vi "VIPM Artifactory Repository.vi"() -> ()   [LabVIEW 2021]
uses:
  Artifactory/Status -- cluster.ctl
  Artifactory/Public Events -- cluster.ctl
  Artifactory/Repository Event -- cluster.ctl
  Artifactory/Actions -- enum.ctl
  Artifactory.VIPM/Artifactory.VIPM.lvclass
  C:/Repositories/francois-normandin-github/Artifactory/lv-src/Artifactory/Artifactory.lvclass
  Artifactory/Artifactory.lvclass/Artifactory.ctl
  Artifactory/Artifactory.lvclass
panel:
  in  "Show in File Explorer":bool
  out "Status":T1
  in  "Download Package":bool
  out "Status Events":string
  in  "Scan":bool
  in  "Update":bool
  in  "Local Packages":i32(listbox)=-1
  out "Local Repository":path
  out "File Path out":path
  in  "File Path":path
  out "Sync'ed Files":path[](array[path])
  in  "Remote Packages":i32(listbox)=-1
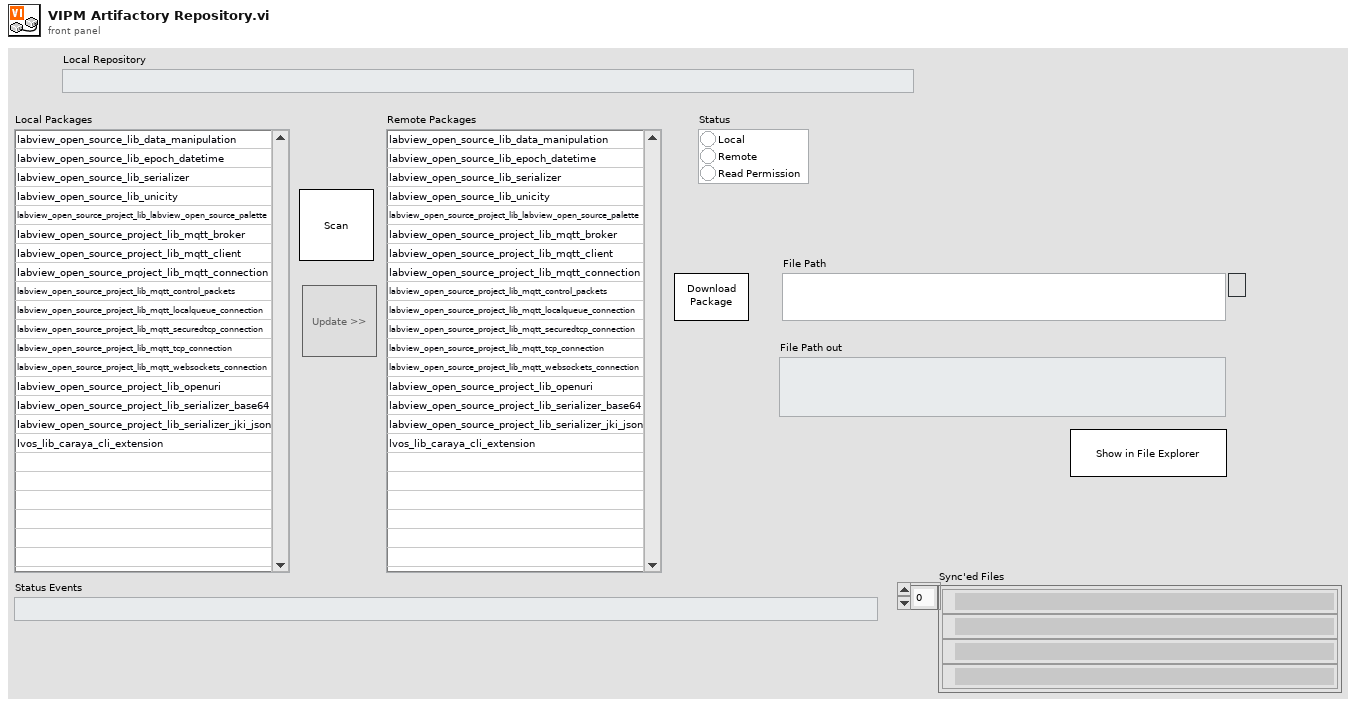
[diagram p1: front panel]
types:
  T1 = typedef "Artifactory.lvclass/Status -- cluster.ctl" = cluster{"Local":bool, "Remote":bool, "Read Permission":bool}
  T2 = typedef "Artifactory.lvclass/Public Events -- cluster.ctl" = cluster{"Action":refnum<user-event>}
  T3 = enum32{"Invalid", "Standard", "Closed", "Hidden", "Minimized", "Maximized"}
  T4 = enum32{"invalid app kind", "Development System", "Run Time System", "Student Edition", "Embedded LabVIEW", "Evaluation", "Custom"}
  T5 = enum8{"Enabled", "Disabled", "Disabled and Grayed Out"}
  T6 = typedef "Artifactory.lvclass/Actions -- enum.ctl" = enum16{"Idle", "Custom Event", "Connecting to Artifactory", "Verifying Permissions", "Listing local repository", "Listing remote repository", "Computing changes", "Uploading file", "Downloading file"}
  T7 = cluster{"Core":cluster{"Current VI Reference":refnum<vi>, "Close Panel on Exit?":bool}, "Artifactory":refnum<class "Artifactory.VIPM.lvclass">, "initialized":bool, "Remote Packages":map{string, string[]}, "Local Packages":map{string, string[]}, "Diff":map{string, string[]}}
  T8 = cluster{"Current VI Reference":refnum<vi>, "Close Panel on Exit?":bool}
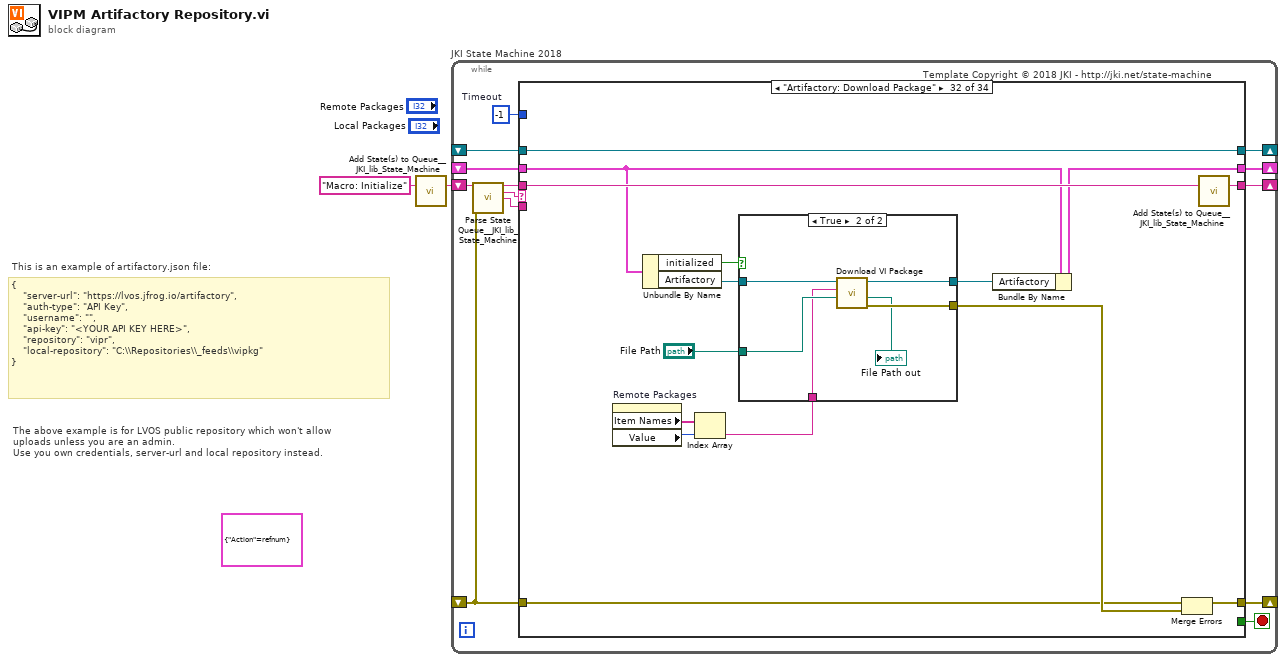
[diagram p0: block diagram]
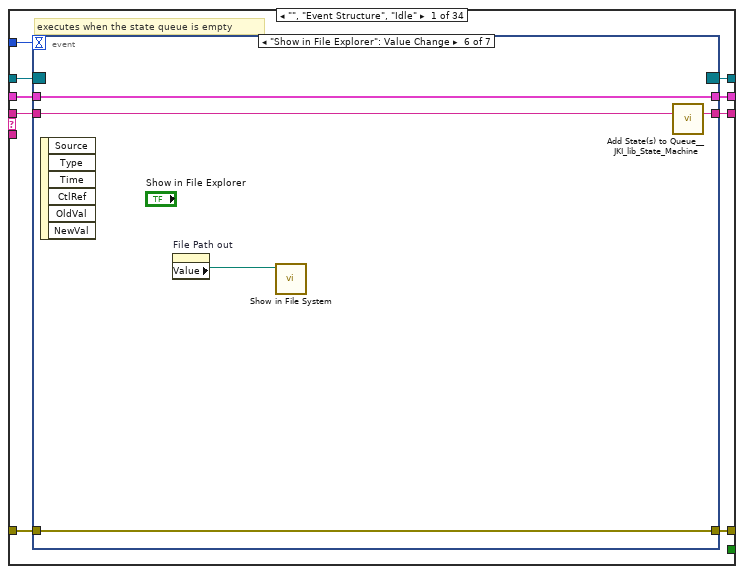
[diagram p2: hidden frame]
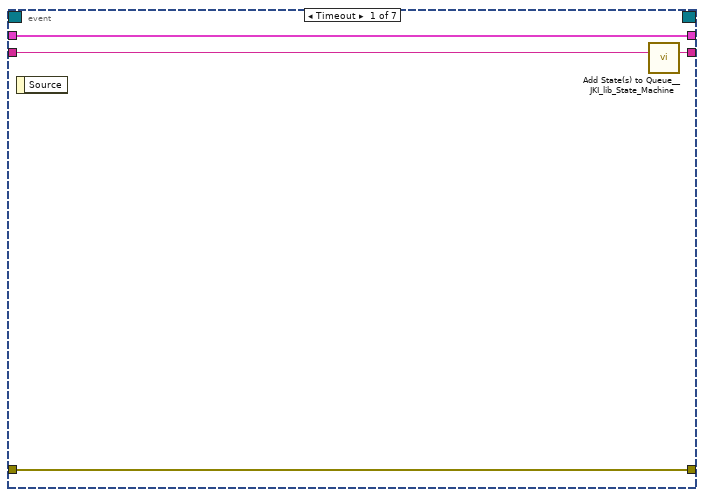
[diagram p3: hidden frame]
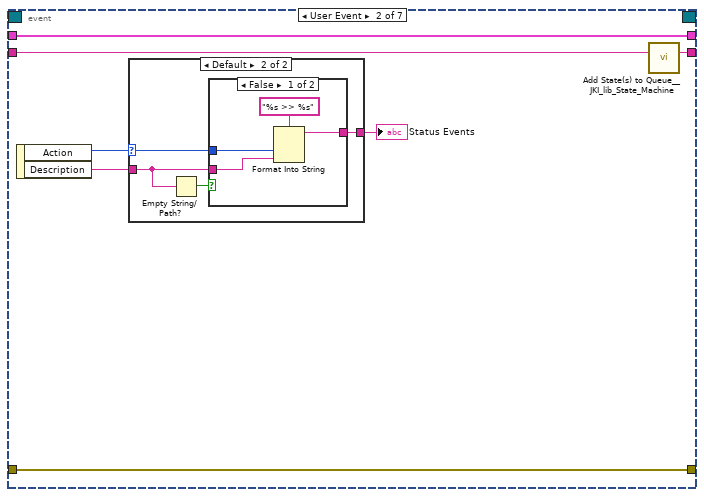
[diagram p4: hidden frame]
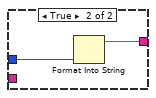
[diagram p6: hidden frame]
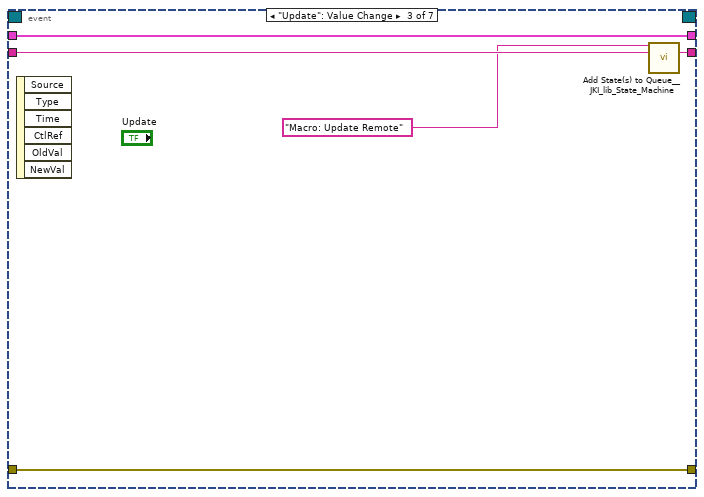
[diagram p7: hidden frame]
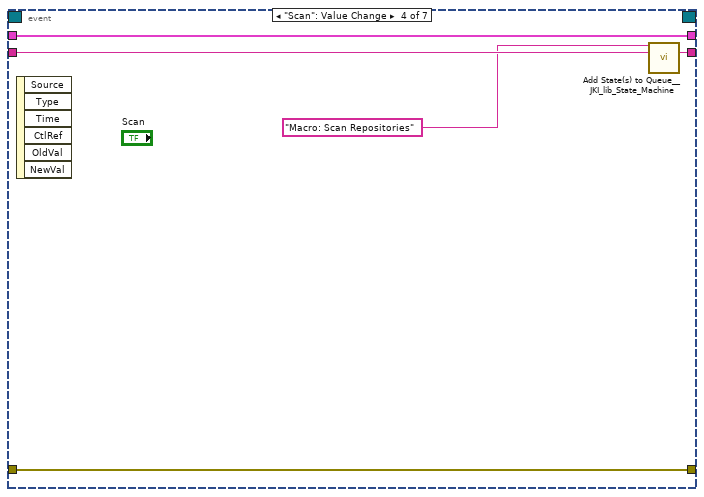
[diagram p8: hidden frame]
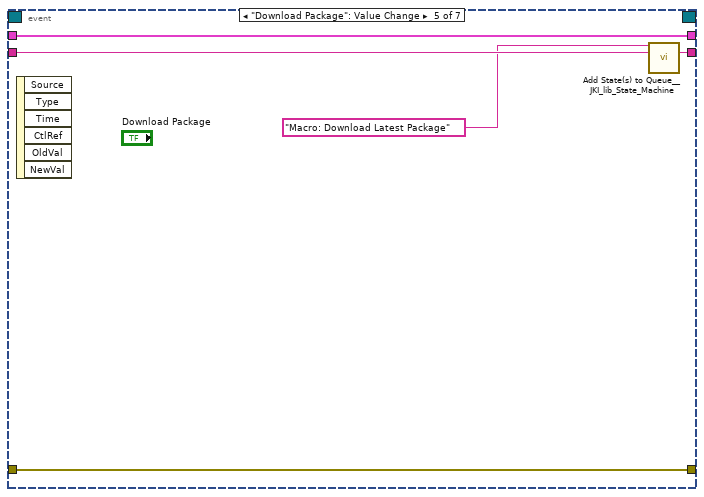
[diagram p9: hidden frame]
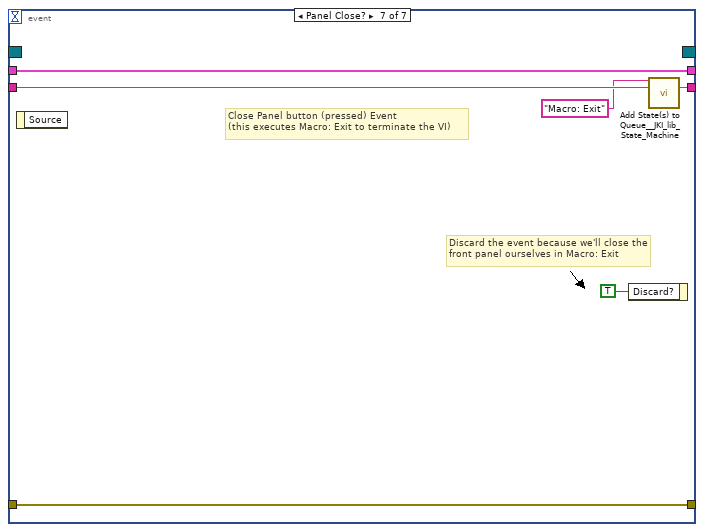
[diagram p10: hidden frame]
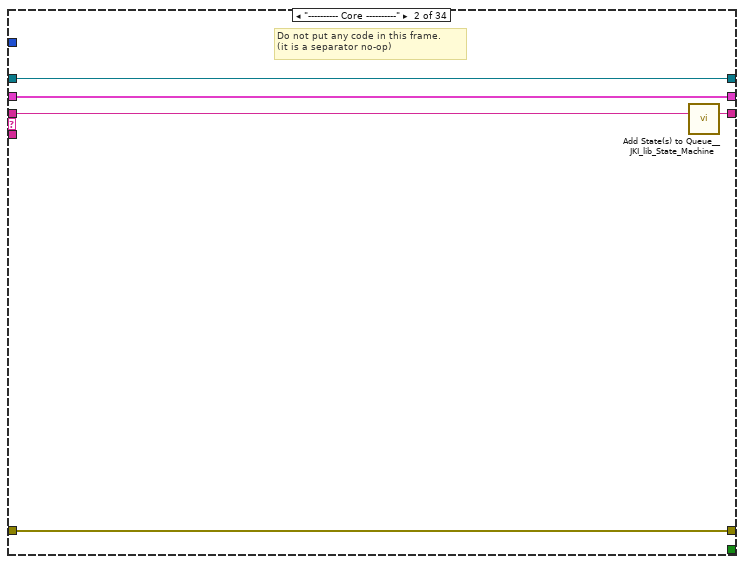
[diagram p11: hidden frame]
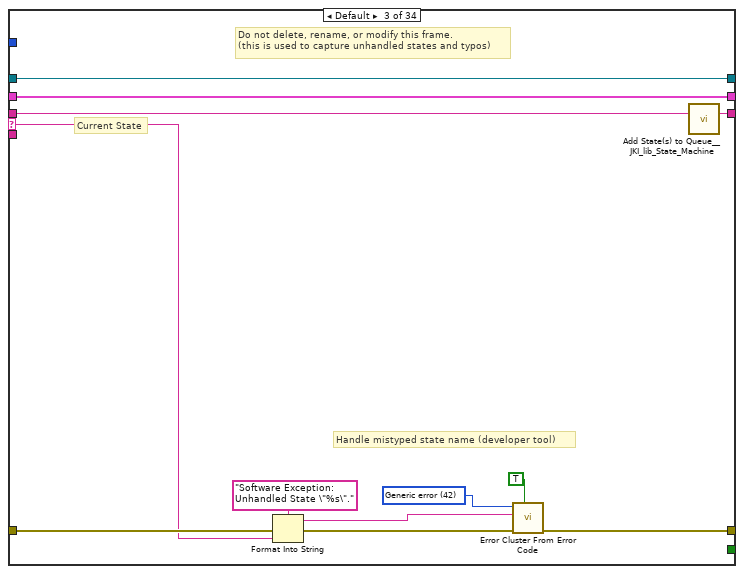
[diagram p12: hidden frame]
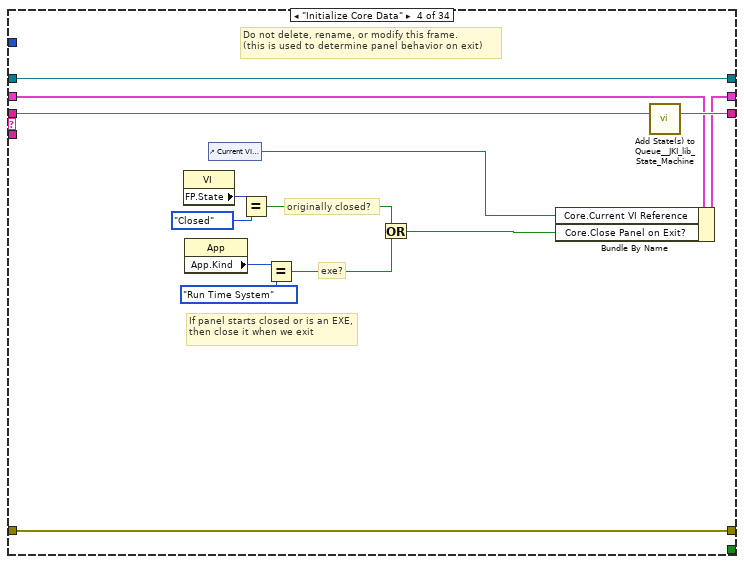
[diagram p13: hidden frame]
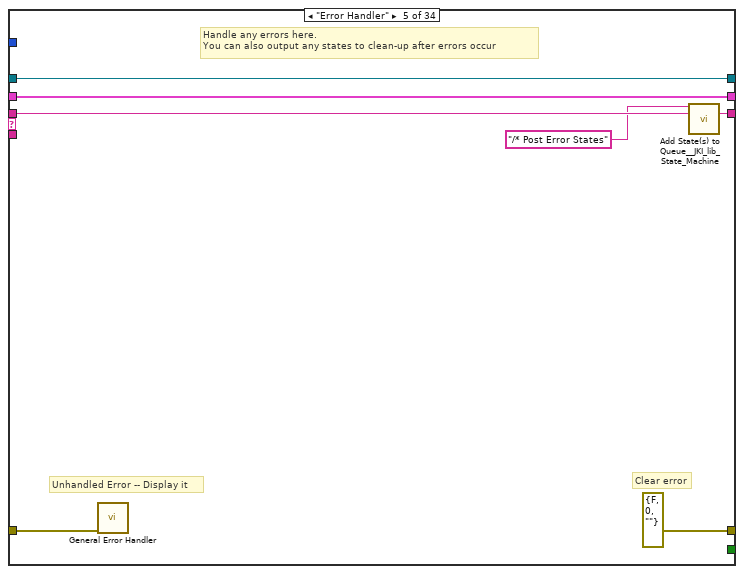
[diagram p14: hidden frame]
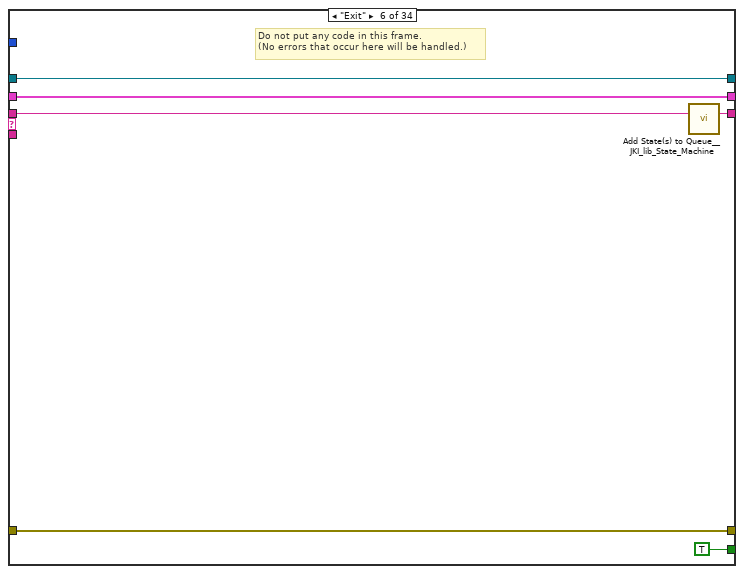
[diagram p15: hidden frame]
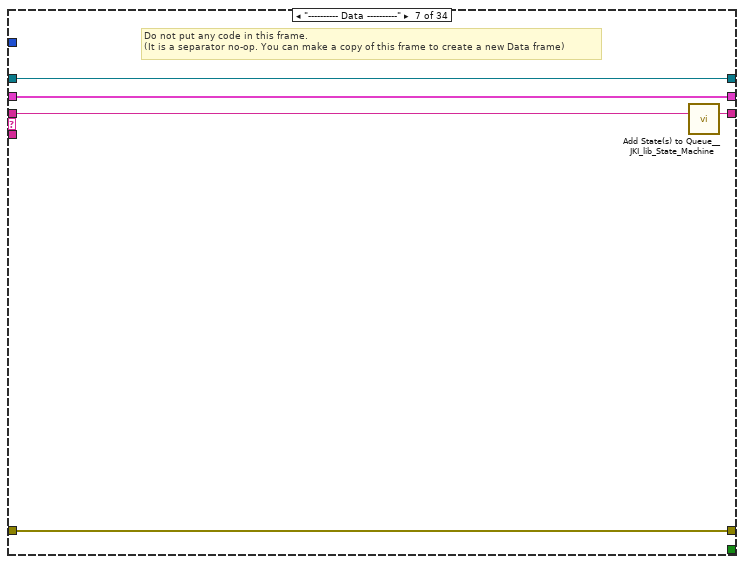
[diagram p16: hidden frame]
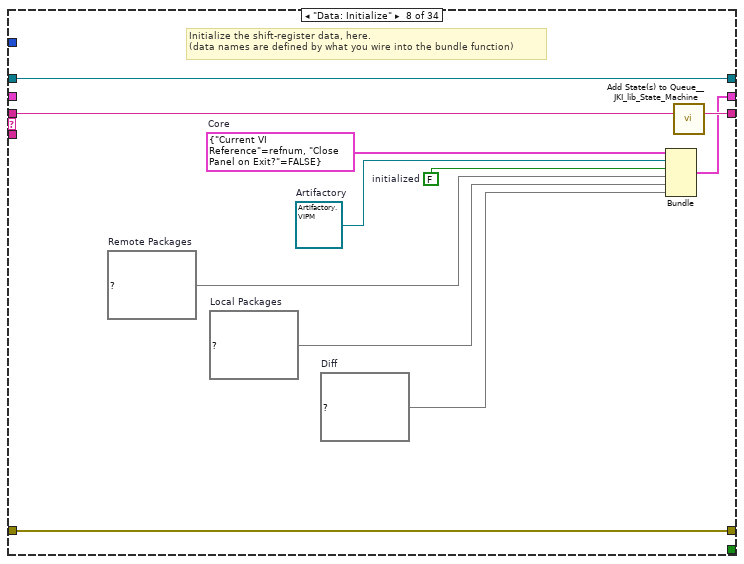
[diagram p17: hidden frame]
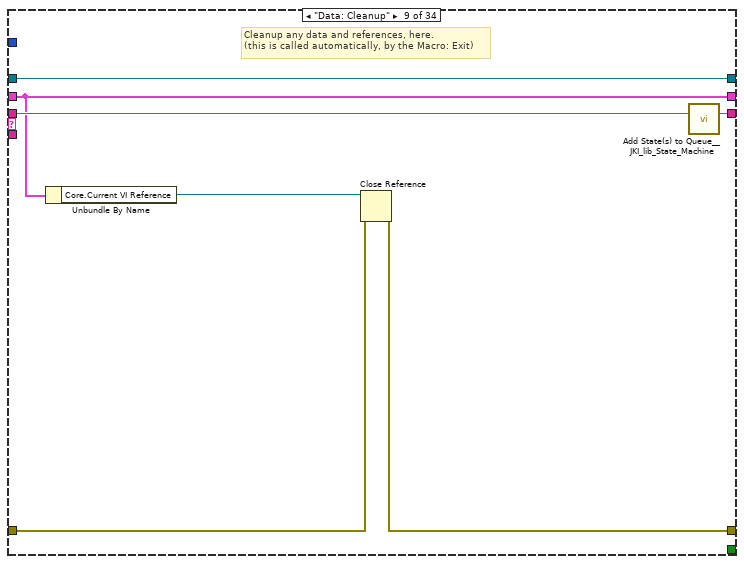
[diagram p18: hidden frame]
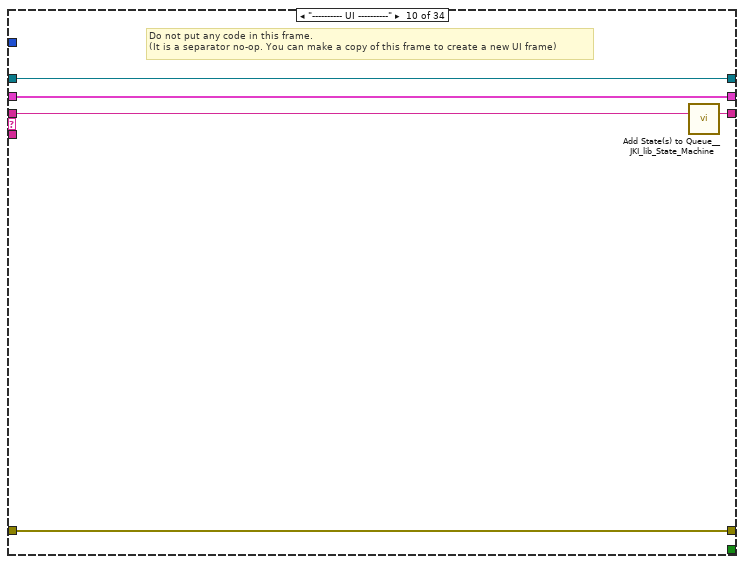
[diagram p19: hidden frame]
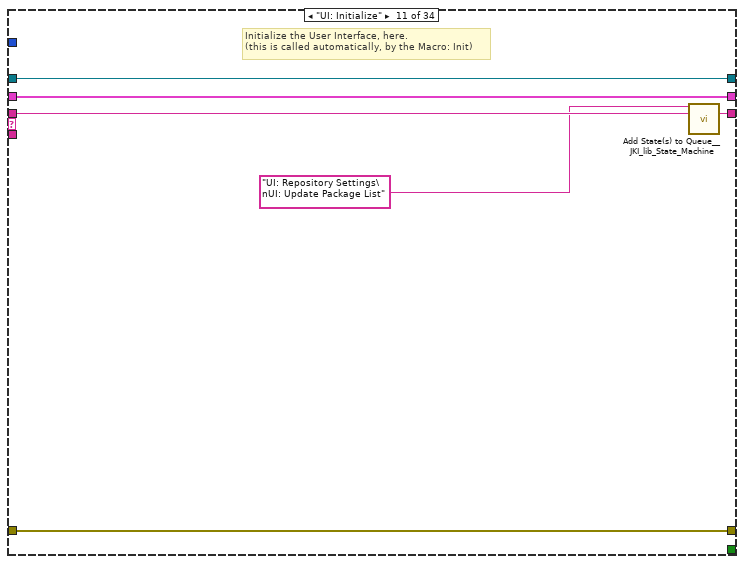
[diagram p20: hidden frame]
diagram:
  (unwired) T2 {"Action"=refnum} ("Public Events")
  # "The above example is for LVOS public repository which won't allow\nuploads unless you are an admin.\nUse you own credentials, server-url and local repository instead."
  # "This is an example of artifactory.json file:"
  # "{\n    \"server-url\": \"https://lvos.jfrog.io/artifactory\",\n\t   \"auth-type\": \"API Key\",\n\t   \"username\": \"\",\n    \"api-key\": \"<YOUR API KEY HERE>\",\n\t   \"repository\": \"vipr\",\n\t   \"local-repository\": \"C:\\\\Repositories\\\\_feeds\\\\vipkg\"\n}"
  n1 = call <vilib>:"Add State(s) to Queue__JKI_lib_State_Machine.vi"("State(s) in (\"\")"="Macro: Initialize") -> ("States Out"=w2:string)  [unwired: 14 in]
  n2 = while "JKI State Machine 2018" {
    shift-right: [w8] -> _
    shift-left: _ -> [w7]
    shift-right: [w11] -> _
    shift-left: _ -> [w5]
    shift-right: [w10] -> _
    shift-left: w2 -> [w12]
    shift-right: [w4] -> _
    shift-left: _ -> [w3]
    stop <- w9 stop-if-true
    w6 = -1  # Timeout
    # "Template Copyright © 2018 JKI - http://jki.net/state-machine"
    n3 = call <vilib>:"Parse State Queue__JKI_lib_State_Machine.vi"("State Queue"=w12, "Error In (no error)"=w5) -> ("Remaining States"=w14:string, "Current State"=w15:string, "Arguments"=w13:string)  [unwired: 11 in]
    n4 = case shown="\"Artifactory: Download Package\"" w15 {
      selector: w15 -> [_ _ w79 _ _ _ _ _ _ _ _ _ _ _ _ _ _ _ _ _ _ _ _ _ _ _ _ _ _ _ _ _ _ _]
      tunnel: w14 -> [w24 w77 w83 w103 w110 w116 w121 w132 w139 w144 w150 w158 w173 w184 w196 w266 w272 w278 w284 w290 w296 w308 w313 w319 w325 w330 w344 w355 w369 w395 w412 w432 w450 w467]
      tunnel: w13 -> [_ _ _ _ _ _ _ _ _ _ _ _ _ w179 w190 _ _ _ _ _ _ _ _ _ _ _ _ _ _ _ _ _ _ _]
      tunnel: w7 -> [w22 w74 w81 w96 w107 w114 w118 _ w134 w141 w148 w154 w170 w182 w192 w263 w269 w275 w281 w287 w293 w305 w310 w316 w322 w327 w341 w352 w366 w392 w409 w429 w447 w464]
      tunnel: [w21 w75 w85 w100 errorcluster {"status"=FALSE, "code"=0, "source"=""} ("error out") w113 w119 w129 w135 w142 w147 w156 w171 w180 w193 w264 w270 w276 w282 w288 w294 w306 w311 w317 w323 w328 w335 w349 w363 w390 w406 w426 w445 w461] -> w11
      tunnel: w5 -> [w20 w75 w84 w100 w106 w113 w119 w129 w136 w142 w147 w156 w171 w181 w194 w264 w270 w276 w282 w288 w294 w306 w311 w317 w323 w328 w338 w348 w362 w389 w405 w425 w444 w460]
      tunnel: [w23 w76 w82 w102 w109 w115 w120 w131 w138 w143 w149 w157 w172 w183 w195 w265 w271 w277 w283 w289 w295 w307 w312 w318 w324 w329 w343 w354 w368 w394 w411 w431 w449 w466] -> w10
      tunnel: [_ _ _ _ _ TRUE _ _ _ _ _ _ _ _ _ _ _ _ _ _ _ _ _ _ _ _ _ _ _ _ _ _ _ _] -> w9
      tunnel: [w19 w74 w81 w101 w107 w114 w118 w130 w134 w141 w148 w154 w170 w182 w192 w263 w269 w275 w281 w287 w293 w305 w310 w316 w322 w327 w342 w353 w367 w393 w410 w430 w448 w465] -> w8
      tunnel: w6 -> [w18 _ _ _ _ _ _ _ _ _ _ _ _ _ _ _ _ _ _ _ _ _ _ _ _ _ _ _ _ _ _ _ _ _]
      tunnel: [w17 w73 w78 w90 w104 w111 w117 w122 w133 w140 w145 w155 w159 w178 w189 w262 w267 w273 w279 w285 w291 w297 w309 w315 w321 w326 w334 w345 w358 w385 w401 w422 w440 w456] -> w4
      tunnel: w3 -> [w16 w73 w78 w90 w104 w111 w117 w122 w133 w140 w145 w155 w159 w178 w189 w262 w267 w273 w279 w285 w291 w297 w309 _ w321 w326 w333 w345 w358 w385 w401 w422 w440 w456]
      frame "", "Event Structure", "Idle" {
        # "executes when the state queue is empty"
        n5 = event shown="[5] \"Show in File Explorer\": Value Change" {
          selector: w16 -> [_ _ _ _ _ _ _]
          dyn-events: [_ _ _ _ _ _ _] -> w17
          timeout: w18 -> [_ _ _ _ _ _ _]
          tunnel: w24 -> [w28 w35 w51 w56 w61 w66 w72]
          tunnel: [w27 w34 w50 w55 w60 w65 w71] -> w23
          tunnel: w22 -> [w25 w32 w48 w53 w58 w63 w69]
          tunnel: [w26 w33 w49 w54 w59 w64 w70] -> w21
          tunnel: w20 -> [w26 w33 w49 w54 w59 w64 w70]
          tunnel: [w25 w32 w48 w53 w58 w63 w69] -> w19
          event Timeout {
            n6 = event-data() -> ()  [unwired: 1 in, 1 out]
            n7 = call <vilib>:"Add State(s) to Queue__JKI_lib_State_Machine.vi"("State(s) in (\"\")"=w28) -> ("States Out"=w27:string)  [unwired: 14 in]
          }
          event User Event {
            n8 = event-data() -> ("Action"=w29:T6, "Description"=w31:string)  [unwired: 1 in]
            n9 = case shown="Default" w29 {
              selector: w29 -> [_ w39]
              tunnel: w31 -> [w36 w38]
              tunnel: [w36 w40] -> w30
              frame "Custom Event" {
              }
              frame Default {
                n10 = Empty String/Path?(string/path=w38) -> (empty?=w37:bool)
                n11 = case shown="False" w37 {
                  tunnel: [w43 w46] -> w40
                  tunnel: w39 -> [w42 w45]
                  tunnel: w38 -> [w41 _]
                  frame False {
                    n12 = Format Into String(format string="%s >> %s", w42, w41) -> (resulting string=w43:string)  [unwired: 2 in, 1 out]
                  }
                  frame True {
                    n13 = Format Into String(w45) -> (resulting string=w46:string)  [unwired: 3 in, 1 out]
                  }
                }
              }
            }
            "Status Events" <- w30
            n14 = call <vilib>:"Add State(s) to Queue__JKI_lib_State_Machine.vi"("State(s) in (\"\")"=w35) -> ("States Out"=w34:string)  [unwired: 14 in]
          }
          event "Update": Value Change {
            n15 = event-data() -> ()  [unwired: 1 in, 6 out]
            n16 = call <vilib>:"Add State(s) to Queue__JKI_lib_State_Machine.vi"("State(s) in Front (\"\")"="Macro: Update Remote", "State(s) in (\"\")"=w51) -> ("States Out"=w50:string)  [unwired: 13 in]
          }
          event "Scan": Value Change {
            n17 = event-data() -> ()  [unwired: 1 in, 6 out]
            n18 = call <vilib>:"Add State(s) to Queue__JKI_lib_State_Machine.vi"("State(s) in Front (\"\")"="Macro: Scan Repositories", "State(s) in (\"\")"=w56) -> ("States Out"=w55:string)  [unwired: 13 in]
          }
          event "Download Package": Value Change {
            n19 = event-data() -> ()  [unwired: 1 in, 6 out]
            n20 = call <vilib>:"Add State(s) to Queue__JKI_lib_State_Machine.vi"("State(s) in Front (\"\")"="Macro: Download Latest Package", "State(s) in (\"\")"=w61) -> ("States Out"=w60:string)  [unwired: 13 in]
          }
          event "Show in File Explorer": Value Change {
            n21 = event-data() -> ()  [unwired: 1 in, 6 out]
            n22 = property on="File Path out" class="Path"() -> ("Value"=w62:path)  [unwired: 2 in, 2 out]
            n23 = call <vilib>:"Show in File System.vi"("file or directory path"=w62) -> ()  [unwired: 10 in, 1 out]
            n24 = call <vilib>:"Add State(s) to Queue__JKI_lib_State_Machine.vi"("State(s) in (\"\")"=w66) -> ("States Out"=w65:string)  [unwired: 14 in]
          }
          event Panel Close? {
            # "Discard the event because we'll close the front panel ourselves in Macro: Exit"
            # "Close Panel button (pressed) Event\n(this executes Macro: Exit to terminate the VI)"
            n25 = event-data() -> ()  [unwired: 1 in, 1 out]
            n26 = event-data("Discard?"=TRUE) -> ()  [unwired: 1 in, 1 out]
            n27 = call <vilib>:"Add State(s) to Queue__JKI_lib_State_Machine.vi"("State(s) in Front (\"\")"="Macro: Exit", "State(s) in (\"\")"=w72) -> ("States Out"=w71:string)  [unwired: 13 in]
          }
        }
      }
      frame "---------- Core ----------" {
        # "Do not put any code in this frame.\n(it is a separator no-op)"
        n28 = call <vilib>:"Add State(s) to Queue__JKI_lib_State_Machine.vi"("State(s) in (\"\")"=w77) -> ("States Out"=w76:string)  [unwired: 14 in]
      }
      frame Default {
        w88 = 42 items=["No error", "Argument error", "Memory is full", "Out of zone", "End of file", "File already open", "Generic file I/O error", "File not found", "File permission error", "Disk is full", "Duplicate path", "Too many files open", "System feature not enabled", "Resource file not found", "Cannot add resource", "Resource not found", "Image not found", "Image memory error", "Pen does not exist", "Config type invalid", "Config token not found", "Config parse error", "Config memory error", "Bad external code format", "Bad external code offset", "External code not present", "Null window", "Destroy window error", "Null menu", "Print aborted", "Bad print record", "Print driver error", "Windows error during printing", "Memory error during printing", "Print dialog error", "Generic print error", "Invalid device refnum", "Device not found", "Device parameter error", "Device unit error", "Cannot open device", "Device call aborted", "Generic error", "Cancelled by user", "Object ID too low", "Object ID too high", "Object not in heap", "Unknown heap", "Unknown object (invalid DefProc)", "Unknown object (DefProc not in table)", "Message out of range", "Invalid (null) method", "Unknown message", "Manager call not supported", "Bad address", "Network operation in progress", "Network operation timed out", "Connection is busy", "Network attribute not supported", "Network error", "Address in use", "System out of memory", "Connection aborted", "Connection refused", "Not connected", "Already connected", "Connection closed", "Initialization error (interapplication manager)", "Bad occurrence", "Wait on unbound occurrence handler", "Occurrence queue overflow", "Datalog type conflict", "Unused", "Unrecognized type (interapplication manager)", "Memory corrupt", "Failed to make temporary DLL", "Old CIN version", "Drag socket not found", "Failed to load drop-object", "Failed to register OLE object", "Failed to release OLE object", "Format specifier type mismatch", "Unknown format specifier", "Too few format specifiers", "Too many format specifiers", "Scan failed", "Newer CIN version", "Error converting to variant", "Runtime menu error", "Password tampered", "Variant attribute not found", "Incompatible variant data type", "Event data is not available", "Event Store is not present", "Occurrence is not found", "Event Queue is not created", "Event info is not available", "Refnum passed is NULL", "Error retrieving Class GUID", "Error retrieving CoClass GUID", "Error retrieving TypeLib GUID.", "Bad built application magic bytes.", "Specific driver is different from the specific driver associated with the Logical Name.", "There is no session opened to the class driver.", "Max Error", "MAX - Error with config objects", "MAX - Error loading configuration", "MAX - Group not supported"]
        # "Current State"
        # "Do not delete, rename, or modify this frame.\n(this is used to capture unhandled states and typos)"
        # "Handle mistyped state name (developer tool)"
        n29 = Format Into String(format string="Software Exception: Unhandled State \"%s\"." ("message"), error in=w84, w79) -> (resulting string=w87:string, error out=w86:errorcluster)  [unwired: 1 in]
        n30 = call <vilib>:"Error Cluster From Error Code.vi"("show call chain? (False)"=TRUE, "error in (no error)"=w86, "error message (\"\")"=w87, "error code (0)"=w88) -> ("error out"=w85:errorcluster)  [unwired: 5 in]
        n31 = call <vilib>:"Add State(s) to Queue__JKI_lib_State_Machine.vi"("State(s) in (\"\")"=w83) -> ("States Out"=w82:string)  [unwired: 14 in]
      }
      frame "Initialize Core Data" {
        # "Do not delete, rename, or modify this frame.\n(this is used to determine panel behavior on exit)"
        # "originally closed?"
        # "exe?"
        # "If panel starts closed or is an EXE, then close it when we exit"
        n32 = property class="VI"() -> ("FP.State"=w93:T3)  [unwired: 2 in, 2 out]
        n33 = property class="App"() -> ("App.Kind"=w99:T4)  [unwired: 2 in, 2 out]
        n34 = control-ref of="Current VI Reference"() -> (w94:refnum<vi>)
        n35 = Equal?(x=w93, y=T3."Closed" ("Front Panel Window:State")) -> (x = y?=w91:bool)
        n36 = Equal?(x=w99, y=T4."Run Time System" ("Application:Kind")) -> (x = y?=w97:bool)
        n37 = Or(x=w91, y=w97) -> (x .or. y?=w95:bool)
        n38 = Bundle By Name(cluster=w96, "Core.Current VI Reference"=w94, "Core.Close Panel on Exit?"=w95) -> (w101:T7)
        n39 = call <vilib>:"Add State(s) to Queue__JKI_lib_State_Machine.vi"("State(s) in (\"\")"=w103) -> ("States Out"=w102:string)  [unwired: 14 in]
      }
      frame "Error Handler" {
        # "Unhandled Error -- Display it"
        # "Handle any errors here.\nYou can also output any states to clean-up after errors occur"
        # "Clear error"
        n40 = call <vilib>:"General Error Handler.vi"("error in (no error)"=w106) -> ()  [unwired: 10 in, 5 out]
        n41 = call <vilib>:"Add State(s) to Queue__JKI_lib_State_Machine.vi"("State(s) in Front (\"\")"="/* Post Error States", "State(s) in (\"\")"=w110) -> ("States Out"=w109:string)  [unwired: 13 in]
      }
      frame "Exit" {
        # "Do not put any code in this frame.\n(No errors that occur here will be handled.)"
        n42 = call <vilib>:"Add State(s) to Queue__JKI_lib_State_Machine.vi"("State(s) in (\"\")"=w116) -> ("States Out"=w115:string)  [unwired: 14 in]
      }
      frame "---------- Data ----------" {
        # "Do not put any code in this frame.\n(It is a separator no-op. You can make a copy of this frame to create a new Data frame)"
        n43 = call <vilib>:"Add State(s) to Queue__JKI_lib_State_Machine.vi"("State(s) in (\"\")"=w121) -> ("States Out"=w120:string)  [unwired: 14 in]
      }
      frame "Data: Initialize" {
        w123 = refnum<class "Artifactory.VIPM.lvclass"> refnum  # Artifactory
        w124 = map{string, string[]} {}  # Diff
        w125 = map{string, string[]} {}  # Local Packages
        w126 = map{string, string[]} {}  # Remote Packages
        w127 = FALSE  # initialized
        w128 = T8 {"Current VI Reference"=refnum, "Close Panel on Exit?"=FALSE}  # Core
        # "Initialize the shift-register data, here.\n(data names are defined by what you wire into the bundle function)"
        n44 = Bundle("Core"=w128, "Artifactory"=w123, "initialized"=w127, "Remote Packages"=w126, "Local Packages"=w125, "Diff"=w124) -> (w130:T7)  [unwired: 1 in]
        n45 = call <vilib>:"Add State(s) to Queue__JKI_lib_State_Machine.vi"("State(s) in (\"\")"=w132) -> ("States Out"=w131:string)  [unwired: 14 in]
      }
      frame "Data: Cleanup" {
        # "Cleanup any data and references, here.\n(this is called automatically, by the Macro: Exit)"
        n46 = Unbundle By Name(w134) -> ("Core.Current VI Reference"=w137:refnum<vi>)
        n47 = Close Reference(reference=w137, error in (no error)=w136) -> (error out=w135:errorcluster)
        n48 = call <vilib>:"Add State(s) to Queue__JKI_lib_State_Machine.vi"("State(s) in (\"\")"=w139) -> ("States Out"=w138:string)  [unwired: 14 in]
      }
      frame "---------- UI ----------" {
        # "Do not put any code in this frame.\n(It is a separator no-op. You can make a copy of this frame to create a new UI frame)"
        n49 = call <vilib>:"Add State(s) to Queue__JKI_lib_State_Machine.vi"("State(s) in (\"\")"=w144) -> ("States Out"=w143:string)  [unwired: 14 in]
      }
      frame "UI: Initialize" {
        # "Initialize the User Interface, here.\n(this is called automatically, by the Macro: Init)"
        n50 = call <vilib>:"Add State(s) to Queue__JKI_lib_State_Machine.vi"("State(s) in Front (\"\")"="UI: Repository Settings\nUI: Update Package List", "State(s) in (\"\")"=w150) -> ("States Out"=w149:string)  [unwired: 13 in]
      }
      frame "UI: Repository Settings" {
        n51 = Unbundle By Name(w154) -> ("Artifactory"=w152:refnum<class "Artifactory.VIPM.lvclass">)
        n52 = call "Read Local Repository.vi"("Artifactory in"=w152) -> ("Local Repository"=→"Local Repository":path)  [unwired: 9 in, 1 out]
        n53 = call-dynamic "Read Status.vi"("Artifactory in"=w152) -> ("Status"=→"Status":T1)  [unwired: 8 in, 2 out]
        n54 = call <vilib>:"Add State(s) to Queue__JKI_lib_State_Machine.vi"("State(s) in (\"\")"=w158) -> ("States Out"=w157:string)  [unwired: 14 in]
      }
      frame "UI: Update Package List" {
        n55 = Unbundle By Name(w170) -> ("Remote Packages"=w169:map{string, string[]}, "Local Packages"=w167:map{string, string[]}, "Diff"=w164:map{string, string[]})
        n56 = for {
          tunnel: w169 -> [w177] mode=indexing
          tunnel: [w176] -> w168 mode=indexing
          n57 = Unbundle By Name(w177) -> ("package_name"=w176:string)
        }
        n58 = for {
          tunnel: w167 -> [w175] mode=indexing
          tunnel: [w174] -> w166 mode=indexing
          n59 = Unbundle By Name(w175) -> ("package_name"=w174:string)
        }
        n60 = Empty Collection?(1:w164) -> (0:w165:bool)
        n61 = Not(x=w165) -> (.not. x?=w163:bool)
        n62 = property on="Local Packages" class="LstBox (strict)"("Item Names"=w166) -> ()  [unwired: 2 in, 2 out]
        n63 = property on="Remote Packages" class="LstBox (strict)"("Item Names"=w168) -> ()  [unwired: 2 in, 2 out]
        n64 = Select(t=T5."Enabled" ("Disabled"), s=w163, f=T5."Disabled and Grayed Out" ("Disabled")) -> (s? t:f=w161:T5)
        n65 = property on="Update" class="Bool"("DisabledEnum"=w161) -> ()  [unwired: 2 in, 2 out]
        n66 = call <vilib>:"Add State(s) to Queue__JKI_lib_State_Machine.vi"("State(s) in (\"\")"=w173) -> ("States Out"=w172:string)  [unwired: 14 in]
      }
      frame "UI: Cursor Set" {
        # "Argument"
        # "Set and Unset Cursor Busy.\n(Usage: \"UI: Cursor Set >> Busy|Idle\")"
        n67 = case shown="\"Idle\", Default" w179 {
          tunnel: w181 -> [w186 w188]
          tunnel: [w185 w187] -> w180
          frame "Idle", Default {
            n68 = call <vilib>:"Unset Busy.vi"("error in (no error)"=w186) -> ("error out"=w185:errorcluster)  [unwired: 10 in]
          }
          frame "Busy" {
            n69 = call <vilib>:"Set Busy.vi"("error in (no error)"=w188) -> ("error out"=w187:errorcluster)  [unwired: 9 in, 1 out]
          }
        }
        n70 = call <vilib>:"Add State(s) to Queue__JKI_lib_State_Machine.vi"("State(s) in (\"\")"=w184) -> ("States Out"=w183:string)  [unwired: 14 in]
      }
      frame "UI: Front Panel State" {
        # "Argument"
        # "Set Front Panel Open or Closed\n(Usage: \"UI: Front Panel State >> Open|Close\")"
        n71 = Unbundle By Name(w192) -> ("Core.Current VI Reference"=w191:refnum<vi>)
        n72 = case shown="\"Open\", \"Standard\", Default" w190 {
          tunnel: w194 -> [w202 w217 w228 w241 w254]
          tunnel: [w204 w218 w230 w243 w256] -> w193
          tunnel: w191 -> [w203 w215 w229 w242 w255]
          frame "Open", "Standard", Default {
            w197 = T3."Standard" ("State")
            n73 = property class="VI"(reference=w203, error in=w202) -> (reference out=w200:refnum<vi>, error out=w201:errorcluster, "FP.State"=w199:T3)
            n74 = Not Equal?(x=w199, y=w197) -> (x != y?=w198:bool)
            n75 = case shown="False" w198 {
              tunnel: [w208 w210] -> w204
              tunnel: w201 -> [w207 w210]
              tunnel: w200 -> [w206 _]
              tunnel: w197 -> [w205 _]
              frame True {
                n76 = invoke class="VI" method="FP.Open"(reference=w206, error in=w207, "Activate"=TRUE, "State"=w205) -> (error out=w208:errorcluster)  [unwired: 1 in, 4 out]
              }
              frame False {
              }
            }
          }
          frame "Close", "Closed" {
            n77 = property class="VI"(reference=w215, error in=w217) -> (reference out=w214:refnum<vi>, error out=w216:errorcluster, "FP.State"=w212:T3)
            n78 = Not Equal?(x=w212, y=T3."Closed" ("Front Panel Window:State")) -> (x != y?=w211:bool)
            n79 = case shown="True" w211 {
              tunnel: [w219 w222] -> w218
              tunnel: w216 -> [w219 w221]
              tunnel: w214 -> [_ w220]
              frame False {
              }
              frame True {
                n80 = invoke class="VI" method="FP.Close"(reference=w220, error in=w221) -> (error out=w222:errorcluster)  [unwired: 1 in, 2 out]
              }
            }
          }
          frame "Hidden", "Hide" {
            w223 = T3."Hidden" ("State")
            n81 = property class="VI"(reference=w229, error in=w228) -> (reference out=w226:refnum<vi>, error out=w227:errorcluster, "FP.State"=w225:T3)
            n82 = Not Equal?(x=w225, y=w223) -> (x != y?=w224:bool)
            n83 = case shown="True" w224 {
              tunnel: [w234 w235] -> w230
              tunnel: w227 -> [w233 w235]
              tunnel: w226 -> [w232 _]
              tunnel: w223 -> [w231 _]
              frame True {
                n84 = invoke class="VI" method="FP.Open"(reference=w232, error in=w233, "State"=w231) -> (error out=w234:errorcluster)  [unwired: 2 in, 4 out]
              }
              frame False {
              }
            }
          }
          frame "Minimize", "Minimized" {
            w236 = T3."Minimized" ("State")
            n85 = property class="VI"(reference=w242, error in=w241) -> (reference out=w239:refnum<vi>, error out=w240:errorcluster, "FP.State"=w238:T3)
            n86 = Not Equal?(x=w238, y=w236) -> (x != y?=w237:bool)
            n87 = case shown="True" w237 {
              tunnel: [w247 w248] -> w243
              tunnel: w240 -> [w246 w248]
              tunnel: w239 -> [w245 _]
              tunnel: w236 -> [w244 _]
              frame True {
                n88 = invoke class="VI" method="FP.Open"(reference=w245, error in=w246, "State"=w244) -> (error out=w247:errorcluster)  [unwired: 2 in, 4 out]
              }
              frame False {
              }
            }
          }
          frame "Maximize", "Maximized" {
            w249 = T3."Maximized" ("State")
            n89 = property class="VI"(reference=w255, error in=w254) -> (reference out=w252:refnum<vi>, error out=w253:errorcluster, "FP.State"=w251:T3)
            n90 = Not Equal?(x=w251, y=w249) -> (x != y?=w250:bool)
            n91 = case shown="True" w250 {
              tunnel: [w260 w261] -> w256
              tunnel: w253 -> [w259 w261]
              tunnel: w252 -> [w258 _]
              tunnel: w249 -> [w257 _]
              frame True {
                n92 = invoke class="VI" method="FP.Open"(reference=w258, error in=w259, "State"=w257) -> (error out=w260:errorcluster)  [unwired: 2 in, 4 out]
              }
              frame False {
              }
            }
          }
        }
        n93 = call <vilib>:"Add State(s) to Queue__JKI_lib_State_Machine.vi"("State(s) in (\"\")"=w196) -> ("States Out"=w195:string)  [unwired: 14 in]
      }
      frame "---------- Macro ----------" {
        # "Do not put any code in this frame.\n(It is a separator no-op. You can make a copy of this frame to create a new Macro frame)"
        n94 = call <vilib>:"Add State(s) to Queue__JKI_lib_State_Machine.vi"("State(s) in (\"\")"=w266) -> ("States Out"=w265:string)  [unwired: 14 in]
      }
      frame "Macro: Initialize" {
        w268 = "Data: Initialize\nInitialize Core Data\nEvents: Register\nUI: Initialize\nUI: Front Panel State >> Open\n\nMacro: Connect to Repository"  # Data: Initialize Initialize Core Data Events: Register UI: Initialize UI: Front Panel State >> Open  Macro: Connect to Repository
        # "Initialization Macro\n(This is called once, when the VI starts)"
        n95 = call <vilib>:"Add State(s) to Queue__JKI_lib_State_Machine.vi"("State(s) in Front (\"\")"=w268, "State(s) in (\"\")"=w272) -> ("States Out"=w271:string)  [unwired: 13 in]
      }
      frame "Macro: Connect to Repository" {
        n96 = call <vilib>:"Add State(s) to Queue__JKI_lib_State_Machine.vi"("State(s) in Front (\"\")"="Artifactory: Initialize\nUI: Repository Settings\nArtifactory: Check Permissions\nUI: Repository Settings\nMacro: Scan Repositories", "State(s) in (\"\")"=w278) -> ("States Out"=w277:string)  [unwired: 13 in]
      }
      frame "Macro: Scan Repositories" {
        n97 = call <vilib>:"Add State(s) to Queue__JKI_lib_State_Machine.vi"("State(s) in Front (\"\")"="Artifactory: List Local Packages\nArtifactory: List Remote Packages\nArtifactory: Diff\nUI: Update Package List", "State(s) in (\"\")"=w284) -> ("States Out"=w283:string)  [unwired: 13 in]
      }
      frame "Macro: Update Remote" {
        n98 = call <vilib>:"Add State(s) to Queue__JKI_lib_State_Machine.vi"("State(s) in Front (\"\")"="Artifactory: Update Remote\nArtifactory: List Remote Packages\nUI: Update Package List\nMacro: Scan Repositories", "State(s) in (\"\")"=w290) -> ("States Out"=w289:string)  [unwired: 13 in]
      }
      frame "Macro: Download Latest Package" {
        n99 = call <vilib>:"Add State(s) to Queue__JKI_lib_State_Machine.vi"("State(s) in Front (\"\")"="Artifactory: Download Package", "State(s) in (\"\")"=w296) -> ("States Out"=w295:string)  [unwired: 13 in]
      }
      frame "Macro: Exit" {
        # "Exit Macro\n(This is called once, when the VI exits)"
        n100 = Unbundle By Name(w305) -> ("Core.Close Panel on Exit?"=w304:bool)
        n101 = Select(t="UI: Front Panel State >> Close", s=w304, f="") -> (s? t:f=w301:string)
        n102 = call <vilib>:"Add State(s) to Queue__JKI_lib_State_Machine.vi"("State(s) in Front (\"\")"="Artifactory: Close", "State(s) in (\"\")"=w301, "State(s) at Back (\"\")"="Events: Unregister\nData: Cleanup\nExit") -> ("States Out"=w299:string)  [unwired: 12 in]
        n103 = call <vilib>:"Add State(s) to Queue__JKI_lib_State_Machine.vi"("State(s) in Front (\"\")"=w299, "State(s) in (\"\")"=w308) -> ("States Out"=w307:string)  [unwired: 13 in]
      }
      frame "---------- Events ----------" {
        n104 = call <vilib>:"Add State(s) to Queue__JKI_lib_State_Machine.vi"("State(s) in (\"\")"=w313) -> ("States Out"=w312:string)  [unwired: 14 in]
      }
      frame "Events: Register" {
        n105 = register-events(T2 {"Action"=refnum} ("Public Events")) -> (reference out=w315:refnum<event-registration>)  [unwired: 2 in, 1 out]
        n106 = call <vilib>:"Add State(s) to Queue__JKI_lib_State_Machine.vi"("State(s) in (\"\")"=w319) -> ("States Out"=w318:string)  [unwired: 14 in]
      }
      frame "Events: Unregister" {
        n107 = Unregister For Events(event registration refnum=w321) -> (error out=w320:errorcluster)  [unwired: 1 in]
        n108 = call <vilib>:"Clear Errors.vi"("error in (no error)"=w320) -> ()  [unwired: 5 in, 2 out]
        n109 = call <vilib>:"Add State(s) to Queue__JKI_lib_State_Machine.vi"("State(s) in (\"\")"=w325) -> ("States Out"=w324:string)  [unwired: 14 in]
      }
      frame "---------- Artifactory ----------" {
        n110 = call <vilib>:"Add State(s) to Queue__JKI_lib_State_Machine.vi"("State(s) in (\"\")"=w330) -> ("States Out"=w329:string)  [unwired: 14 in]
      }
      frame "Artifactory: Initialize" {
        n111 = call "Connect to Artifactory.vi"("Artifactory in"=refnum<class "Artifactory.VIPM.lvclass"> refnum ("Artifactory.VIPM.lvclass"), "error in (no error)"=w338, "repository path"="vipr", "server-uri"="https://lvos.jfrog.io/artifactory") -> ("error out"=w335:errorcluster, "Public Events"=w331:T2, "Artifactory out"=w332:refnum<class "Artifactory.VIPM.lvclass">)  [unwired: 5 in]
        n112 = register-events(reference=w333, w331) -> (reference out=w334:refnum<event-registration>)  [unwired: 1 in, 1 out]
        n113 = Not(x=w335) -> (.not. x?=w340:bool)
        n114 = Bundle By Name(cluster=w341, "Artifactory"=w332, "initialized"=w340) -> (w342:T7)
        n115 = call <vilib>:"Add State(s) to Queue__JKI_lib_State_Machine.vi"("State(s) in (\"\")"=w344) -> ("States Out"=w343:string)  [unwired: 14 in]
      }
      frame "Artifactory: Close" {
        n116 = Unbundle By Name(w352) -> ("initialized"=w347:bool, "Artifactory"=w351:refnum<class "Artifactory.VIPM.lvclass">)
        n117 = case shown="True" w347 {
          tunnel: w351 -> [_ w357]
          tunnel: [_ w356] -> w350
          frame False {
          }
          frame True {
            n118 = call "Close Artifactory.vi"("Artifactory in"=w357) -> ("error out"=w356:errorcluster)  [unwired: 9 in, 1 out]
          }
        }
        n119 = Merge Errors(w348, w350) -> (w349:errorcluster)
        n120 = Bundle By Name(cluster=w352, "Artifactory"=refnum<class "Artifactory.VIPM.lvclass"> refnum) -> (w353:T7)
        n121 = call <vilib>:"Add State(s) to Queue__JKI_lib_State_Machine.vi"("State(s) in (\"\")"=w355) -> ("States Out"=w354:string)  [unwired: 14 in]
      }
      frame "Artifactory: List Remote Packages" {
        n122 = Unbundle By Name(w366) -> ("initialized"=w361:bool, "Artifactory"=w365:refnum<class "Artifactory.VIPM.lvclass">)
        n123 = case shown="True" w361 {
          tunnel: w365 -> [w370 w373]
          tunnel: [_ w376] -> w364
          tunnel: [w370 w377] -> w360
          tunnel: [_ w375] -> w359
          frame False {
          }
          frame True {
            n124 = call-dynamic "Verify Remote VIPM Repository.vi"("Artifactory.VIPM in"=w373) -> ("error out"=w372:errorcluster, "Repository exists"=w371:bool, "Artifactory.VIPM out"=w374:refnum<class "Artifactory.VIPM.lvclass">)  [unwired: 7 in, 1 out]
            n125 = case shown="True" w371 {
              tunnel: [w379 w384] -> w377
              tunnel: [w378 w383] -> w376
              tunnel: [_ w382] -> w375
              tunnel: w374 -> [w379 w381]
              tunnel: w372 -> [w378 w380]
              frame False {
              }
              frame True {
                n126 = call "Discover Remote Packages.vi"("error in (no error)"=w380, "Artifactory.VIPM in"=w381) -> ("error out"=w383:errorcluster, "Remote Packages"=w382:map{string, string[]}, "Artifactory.VIPM out"=w384:refnum<class "Artifactory.VIPM.lvclass">)  [unwired: 7 in]
              }
            }
          }
        }
        n127 = Bundle By Name(cluster=w366, "Artifactory"=w360, "Remote Packages"=w359) -> (w367:T7)
        n128 = Merge Errors(w362, w364) -> (w363:errorcluster)
        n129 = call <vilib>:"Add State(s) to Queue__JKI_lib_State_Machine.vi"("State(s) in (\"\")"=w369) -> ("States Out"=w368:string)  [unwired: 14 in]
      }
      frame "Artifactory: Check Permissions" {
        n130 = Unbundle By Name(w392) -> ("initialized"=w388:bool, "Artifactory"=w391:refnum<class "Artifactory.VIPM.lvclass">)
        n131 = case shown="True" w388 {
          tunnel: w391 -> [w396 w400]
          tunnel: [w396 w399] -> w387
          tunnel: [_ w397] -> _
          tunnel: [_ w398] -> w386
          frame False {
          }
          frame True {
            n132 = call-dynamic "Verify Remote VIPM Repository.vi"("Artifactory.VIPM in"=w400) -> ("error out"=w398:errorcluster, "Read Permission"=w397:bool, "Artifactory.VIPM out"=w399:refnum<class "Artifactory.VIPM.lvclass">)  [unwired: 7 in, 1 out]
          }
        }
        n133 = Bundle By Name(cluster=w392, "Artifactory"=w387) -> (w393:T7)
        n134 = Merge Errors(w389, w386) -> (w390:errorcluster)
        n135 = call <vilib>:"Add State(s) to Queue__JKI_lib_State_Machine.vi"("State(s) in (\"\")"=w395) -> ("States Out"=w394:string)  [unwired: 14 in]
      }
      frame "Artifactory: Diff" {
        n136 = Unbundle By Name(w409) -> ("initialized"=w404:bool, "Artifactory"=w408:refnum<class "Artifactory.VIPM.lvclass">)
        n137 = case shown="True" w404 {
          tunnel: w408 -> [w413 w417]
          tunnel: [_ w414] -> w407
          tunnel: [w413 w416] -> w403
          tunnel: [_ w415] -> w402
          frame False {
          }
          frame True {
            n138 = call "Diff Remote-Local.vi"("Artifactory.VIPM in"=w417) -> ("error out"=w414:errorcluster, "DIff"=w415:map{string, string[]}, "Artifactory.VIPM out"=w416:refnum<class "Artifactory.VIPM.lvclass">)  [unwired: 7 in, 1 out]
          }
        }
        n139 = Bundle By Name(cluster=w409, "Artifactory"=w403, "Diff"=w402) -> (w410:T7)
        n140 = Merge Errors(w405, w407) -> (w406:errorcluster)
        n141 = call <vilib>:"Add State(s) to Queue__JKI_lib_State_Machine.vi"("State(s) in (\"\")"=w412) -> ("States Out"=w411:string)  [unwired: 14 in]
      }
      frame "Artifactory: Download Package" {
        n142 = property on="Remote Packages" class="LstBox (strict)"() -> ("Item Names"=w420:string[], "Value"=w419:i32)  [unwired: 2 in, 2 out]
        n143 = Unbundle By Name(w429) -> ("initialized"=w424:bool, "Artifactory"=w428:refnum<class "Artifactory.VIPM.lvclass">)
        n144 = Index Array(array=w420, index=w419) -> (element=w418:string)
        n145 = case shown="True" w424 {
          tunnel: w428 -> [w433 w439]
          tunnel: [_ w437] -> w427
          tunnel: [w433 w438] -> w423
          tunnel: "File Path" -> [_ w436]
          tunnel: w418 -> [_ w435]
          frame False {
          }
          frame True {
            n146 = call "Download VI Package.vi"("File Path"=w436, "Package Name"=w435, "Artifactory.VIPM"=w439) -> ("error out"=w437:errorcluster, "File Path out"=→"File Path out":path, "Artifactory.VIPM out"=w438:refnum<class "Artifactory.VIPM.lvclass">)  [unwired: 6 in]
          }
        }
        n147 = Bundle By Name(cluster=w429, "Artifactory"=w423) -> (w430:T7)
        n148 = Merge Errors(w425, w427) -> (w426:errorcluster)
        n149 = call <vilib>:"Add State(s) to Queue__JKI_lib_State_Machine.vi"("State(s) in (\"\")"=w432) -> ("States Out"=w431:string)  [unwired: 14 in]
      }
      frame "Artifactory: Update Remote" {
        n150 = Unbundle By Name(w447) -> ("initialized"=w443:bool, "Artifactory"=w446:refnum<class "Artifactory.VIPM.lvclass">)
        n151 = case shown="True" w443 {
          tunnel: w446 -> [w451 w455]
          tunnel: [w451 w454] -> w442
          tunnel: [_ w453] -> w441
          frame False {
          }
          frame True {
            n152 = call "Update Packages (Diff).vi"("Artifactory.VIPM in"=w455) -> ("error out"=w453:errorcluster, "Sync'ed Files"=→"Sync'ed Files":path[], "Artifactory.VIPM out"=w454:refnum<class "Artifactory.VIPM.lvclass">)  [unwired: 8 in]
          }
        }
        n153 = Bundle By Name(cluster=w447, "Artifactory"=w442) -> (w448:T7)
        n154 = Merge Errors(w444, w441) -> (w445:errorcluster)
        n155 = call <vilib>:"Add State(s) to Queue__JKI_lib_State_Machine.vi"("State(s) in (\"\")"=w450) -> ("States Out"=w449:string)  [unwired: 14 in]
      }
      frame "Artifactory: List Local Packages" {
        n156 = Unbundle By Name(w464) -> ("initialized"=w459:bool, "Artifactory"=w463:refnum<class "Artifactory.VIPM.lvclass">)
        n157 = case shown="True" w459 {
          tunnel: w463 -> [w468 w472]
          tunnel: [_ w469] -> w462
          tunnel: [w468 w471] -> w458
          tunnel: [_ w470] -> w457
          frame False {
          }
          frame True {
            n158 = call "Discover Local Packages.vi"("Artifactory.VIPM in"=w472) -> ("error out"=w469:errorcluster, "Local Packages"=w470:map{string, string[]}, "Artifactory.VIPM out"=w471:refnum<class "Artifactory.VIPM.lvclass">)  [unwired: 8 in]
          }
        }
        n159 = Bundle By Name(cluster=w464, "Artifactory"=w458, "Local Packages"=w457) -> (w465:T7)
        n160 = Merge Errors(w460, w462) -> (w461:errorcluster)
        n161 = call <vilib>:"Add State(s) to Queue__JKI_lib_State_Machine.vi"("State(s) in (\"\")"=w467) -> ("States Out"=w466:string)  [unwired: 14 in]
      }
    }
  }
